vi "DLLPathFromAPPDir.vi"() -> (0 "error out":errorcluster, 3 "DLLPath":path)   [LabVIEW 2010]
doc: "Attemps to load pdlm_lib.dll DLL from subfolder of application path"
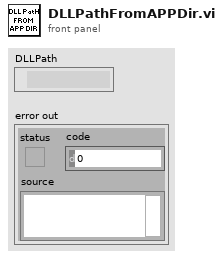
[diagram p1: front panel]
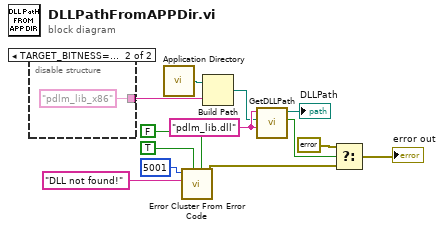
[diagram p0: block diagram]
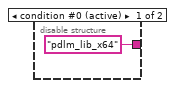
[diagram p2: hidden frame]
diagram:
  w7 = "pdlm_lib.dll" ("DllName_64bit")
  n1 = disable-structure shown="TARGET_BITNESS==32" {
    disable-tunnel: ["pdlm_lib_x64" "pdlm_lib_x86"] -> w8
    frame condition #0 (active) {
    }
    frame condition #1 {
    }
  }
  n2 = call <vilib>:"Application Directory.vi"() -> ("Application Directory"=w6:path)
  n3 = call <vilib>:"Error Cluster From Error Code.vi"("is warning? (False)"=FALSE, "show call chain? (False)"=TRUE, "error message (\"\")"="DLL not found!" ("error message (\"\")"), "error code (0)"=5001) -> ("error out"=w12:errorcluster)  [unwired: 5 in]
  n4 = Build Path(base path=w6, name or relative path=w8) -> (appended path=w5:path)
  n5 = call "GetDLLPath.vi"("DllName_32bit"=w7, "PathToDLL"=w5, "DllName_64bit"=w7) -> ("file exists?"=w11:bool, "DLLPath"=→"DLLPath":path)  [unwired: 7 in]
  n6 = Select(t=errorcluster {"status"=FALSE, "code"=0, "source"=""} ("error in (no error)"), s=w11, f=w12) -> (s? t:f=→"error out":errorcluster)
